vi "Read Font Setups.vi"(4 "error in (no error)":errorcluster, 6 "Owner Name":string, 7 "Config Data in":refnum<class "Config Data.lvclass">) -> (0 "error out":errorcluster, 1 "Control Names":string[](array[string]), 2 "Font Parameters":cluster{T1[]}[](array[cluster]), 3 "Config Data out":refnum<class "Config Data.lvclass">)   [LabVIEW 2015, in "Config Data.lvlib" / "Config Data.lvclass"]
uses:
  Config Data.lvclass
  Display Properties Manager/_typedefs/Font Parameters.ctl
  Display Properties Manager/_typedefs/Control Component to Set.ctl
  Display Properties Manager/_typedefs/Font Setting Definition.ctl
  Display Properties Manager/Display Properties Manager.lvlib
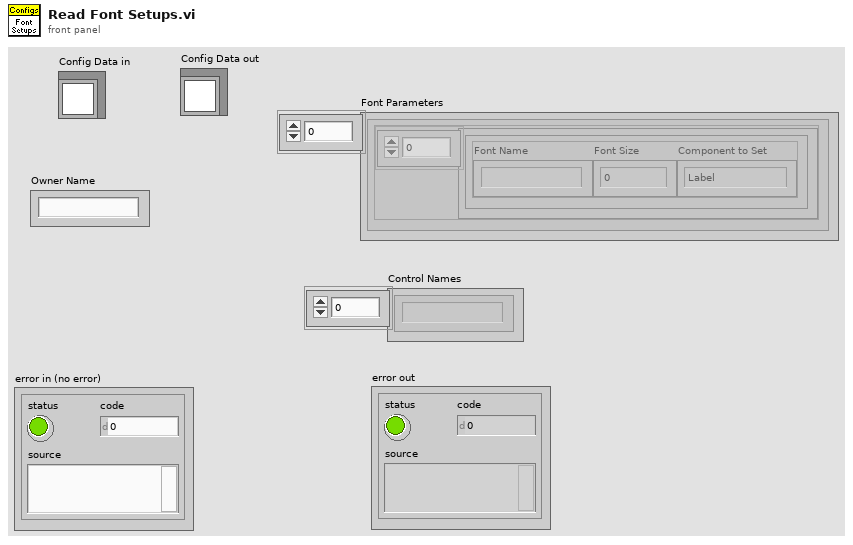
[diagram p1: front panel]
types:
  T1 = typedef "Display Properties Manager.lvlib/Font Parameters.ctl" = cluster{"Font Name":string, "Font Size":u32, "Component to Set":T2}
  T2 = typedef "Display Properties Manager.lvlib/Control Component to Set.ctl" = enum16{"Label", "Caption", "Contents"}
  T3 = typedef "Display Properties Manager.lvlib/Font Setting Definition.ctl" = cluster{"Control Name":string, "Font Parameters":T1}
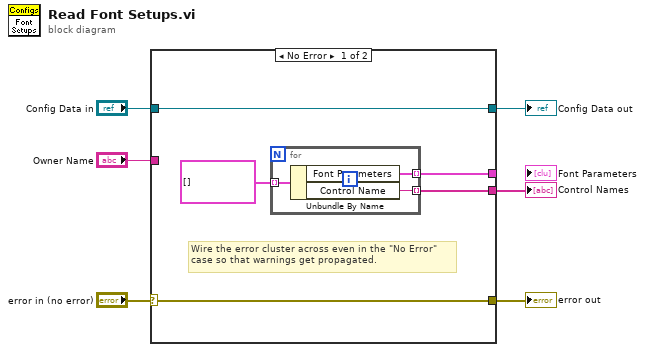
[diagram p0: block diagram]
diagram:
  n1 = case shown="No Error" "error in (no error)" {
    selector: "error in (no error)" -> [w10 w16]
    tunnel: [w10 w16] -> w5
    tunnel: [w11 w15] -> w3
    tunnel: "Config Data in" -> [w11 w15]
    tunnel: "Owner Name" -> [_ _]
    tunnel: [w8 _] -> _
    tunnel: [w7 _] -> w1
    frame No Error {
      # "Wire the error cluster across even in the \"No Error\"\ncase so that warnings get propagated."
      n2 = for {
        tunnel: T3[] [] -> [w14] mode=indexing
        tunnel: [w13] -> w8 mode=indexing
        tunnel: [w12] -> w7 mode=indexing
        n3 = Unbundle By Name(w14) -> ("Font Parameters"=w13:T1, "Control Name"=w12:string)
      }
    }
    frame Error {
    }
  }
  "error out" <- w5
  "Config Data out" <- w3
  "Control Names" <- w1
